vi "mmToUm.vi"(1 "distance (mm)":dbl) -> (0 "distance (um)":dbl)   [LabVIEW 2015]
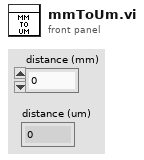
[diagram p1: front panel]
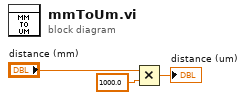
[diagram p0: block diagram]
diagram:
  n1 = Multiply(x="distance (mm)", y=1000.0) -> (x*y=→"distance (um)":dbl)
